vi "Exit.vi"(7 "Enum":enum16{"Initial", "Read", "Write"}(ring)=enum."Read", 10 "ExitIn":bool) -> (2 "ExitOut":bool)   [LabVIEW 2019, in "Commonly VI.lvlib"]
uses:
  Commonly VI.lvlib
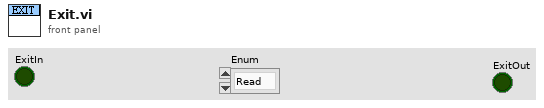
[diagram p1: front panel]
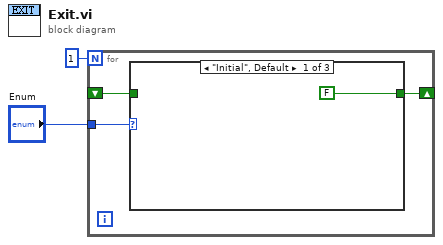
[diagram p0: block diagram]
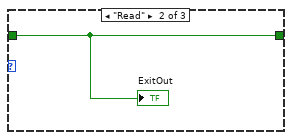
[diagram p2: hidden frame]
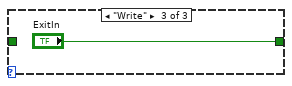
[diagram p3: hidden frame]
diagram:
  n1 = for {
    N: 1 -> [_]
    tunnel: "Enum" -> [w5]
    shift-right: [w4] -> _
    shift-left: _ -> [w3]
    n2 = case shown="\"Initial\", Default" w5 {
      tunnel: [FALSE w7 "ExitIn"] -> w4
      tunnel: w3 -> [_ w7 _]
      frame "Initial", Default {
      }
      frame "Read" {
        "ExitOut" <- w7
      }
      frame "Write" {
      }
    }
  }
